vi "xijk_combined_search_in_file.vi"(6 "file path in":path, 7 "index (col)":i32, 8 "error in (no error)":errorcluster, 9 "channel":string, 10 "search input":string="#BS1", 11 "search 2D array":string[][](array[string])) -> (0 "error out":errorcluster, 3 "file path out":path)   [LabVIEW 2010, in "xijk_combined_file.lvlib"]
uses:
  xijk_combined_file.lvlib
  <vilib>/Utility/file.llb/Write To Spreadsheet File (string).vi
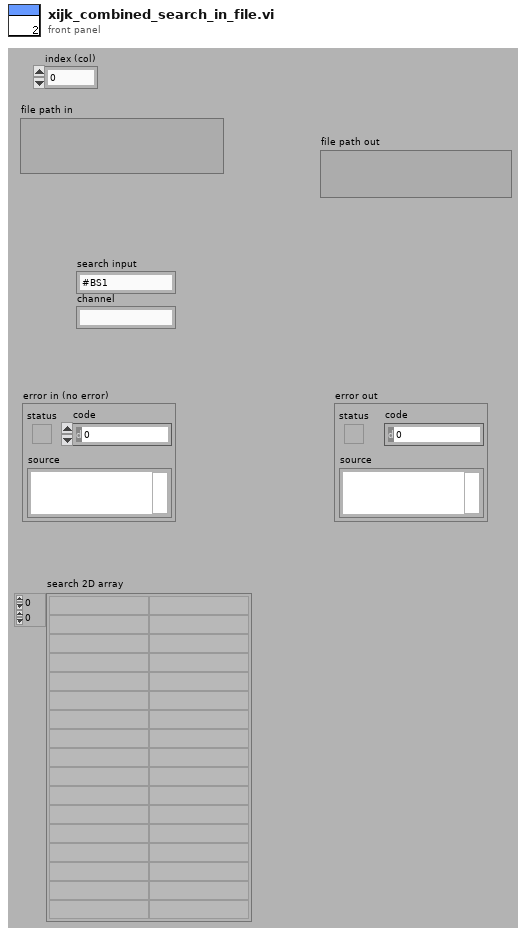
[diagram p1: front panel]
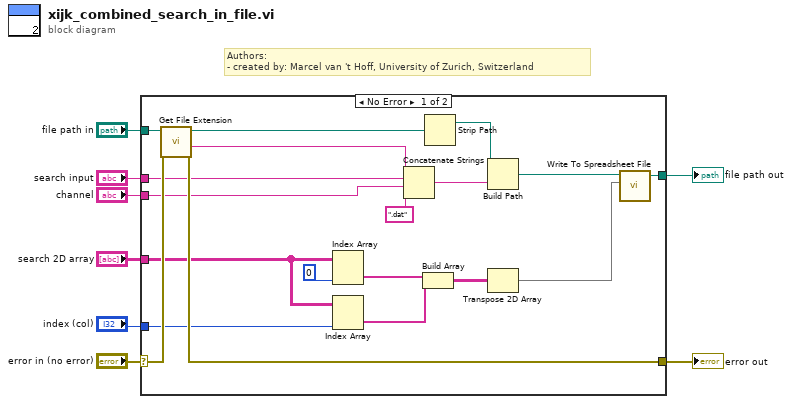
[diagram p0: block diagram]
diagram:
  # "Authors: \n- created by: Marcel van 't Hoff, University of Zurich, Switzerland"
  n1 = case shown="No Error" "error in (no error)" {
    selector: "error in (no error)" -> [w17 w29]
    tunnel: [w26 w28] -> w8
    tunnel: "file path in" -> [w19 w28]
    tunnel: [w16 w29] -> w5
    tunnel: "search 2D array" -> [w15 _]
    tunnel: "index (col)" -> [w14 _]
    tunnel: "search input" -> [w13 _]
    tunnel: "channel" -> [w12 _]
    frame No Error {
      n2 = call <vilib>:"Get File Extension.vi"("error in (no error)"=w17, "file"=w19) -> ("error out"=w16:errorcluster, "filename without extension"=w18:string, "dup file"=w11:path)  [unwired: 6 in, 1 out]
      n3 = Index Array(array=w15, index (col)=0 ("disabled index (col)")) -> (element=w23:string[])  [unwired: 1 in]
      n4 = Index Array(array=w15, index (col)=w14) -> (element=w22:string[])  [unwired: 1 in]
      n5 = Concatenate Strings(w18, w13, w12, ".dat" ("string")) -> (w10:string)
      n6 = Build Array(w23, w22) -> (w21:string[][])
      n7 = Strip Path(path=w11) -> (stripped path=w9:path)  [unwired: 1 out]
      n8 = Build Path(base path=w9, name or relative path=w10) -> (appended path=w27:path)
      n9 = Transpose 2D Array(2D array=w21) -> (transposed array=w20:string[][])
      n10 = call-poly <vilib>:"Write To Spreadsheet File.vi"("2D data"=w20, "file path (dialog if empty)"=w27) -> ("new file path (Not A Path if cancelled)"=w26:path)  [unwired: 6 in]
    }
    frame Error {
    }
  }
  "file path out" <- w8
  "error out" <- w5
